vi "4Decembre2016.vi"() -> ()   [LabVIEW 2014]
panel:
  out "Partie 2 ID":i32
  out "Partie 2":string[](array[string])
  out "Partie 1":i32
  out "CharPlusLettre":string[](array[string])
  out "CharPlusNombre":i32[](array[numeric])
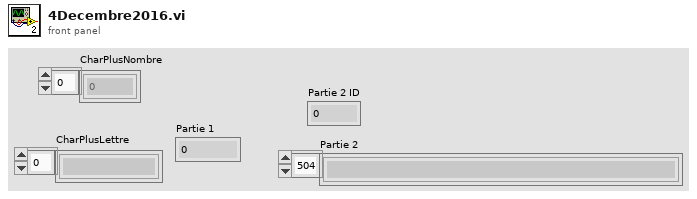
[diagram p1: front panel]
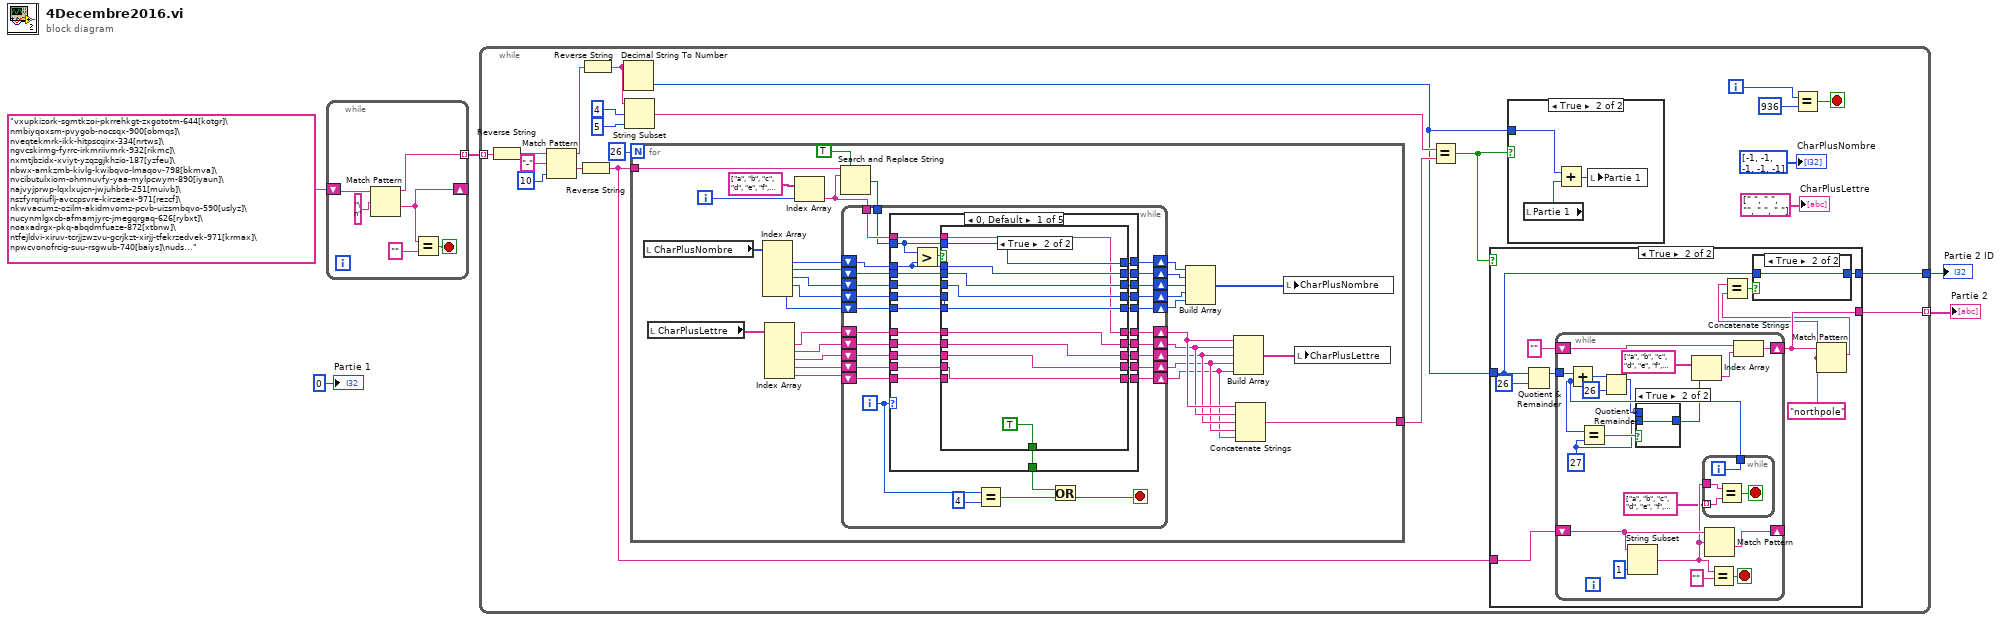
[diagram p0: block diagram]
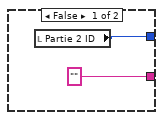
[diagram p2: hidden frame]
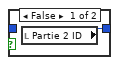
[diagram p3: hidden frame]
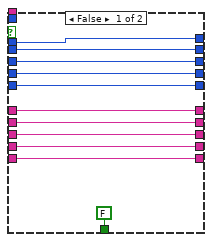
[diagram p6: hidden frame]
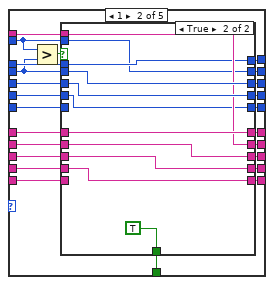
[diagram p7: hidden frame]
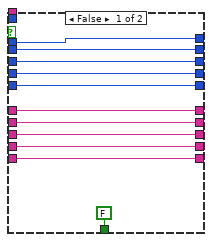
[diagram p8: hidden frame]
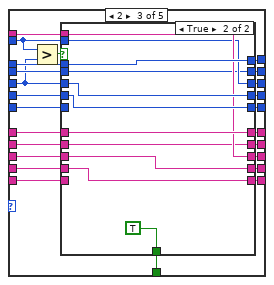
[diagram p9: hidden frame]
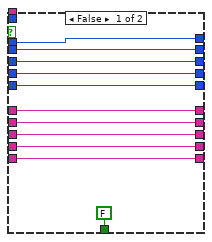
[diagram p10: hidden frame]
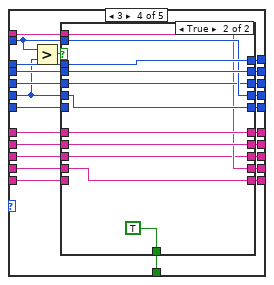
[diagram p11: hidden frame]
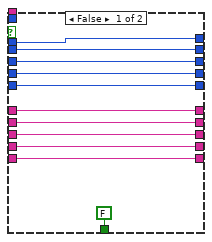
[diagram p12: hidden frame]
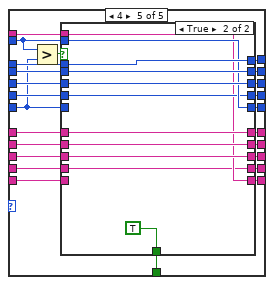
[diagram p13: hidden frame]
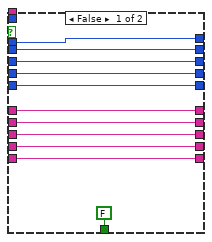
[diagram p14: hidden frame]
diagram:
  n1 = while {
    shift-right: [w8] -> _
    shift-left: "vxupkizork-sgmtkzoi-pkrrehkgt-zxgototm-644[kotgr]\nmbiyqoxsm-pvygob-nocsqx-900[obmqs]\nveqtekmrk-ikk-hitpscqirx-334[nrtws]\ngvcskirmg-fyrrc-irkmriivmrk-932[rikmc]\nxmtjbzidx-xviyt-yzqzgjkhzio-187[yzfeu]\nbwx-amkzmb-kivlg-kwibqvo-lmaqov-798[bkmva]\nvcibutulxiom-ohmnuvfy-yaa-mylpcwym-890[iyaun]\najvyjprwp-lqxlxujcn-jwjuhbrb-251[muivb]\nszfyrqriuflj-avccpsvre-kirzezex-971[rezcf]\nkwvacumz-ozilm-akidmvomz-pcvb-uizsmbqvo-590[uslyz]\nucynmlgxcb-afmamjyrc-jmegqrgaq-626[rybxt]\noaxadrgx-pkq-abqdmfuaze-872[xtbnw]\ntfejldvi-xiruv-tcrjjzwzvu-gcrjkzt-xirjj-tfekrzedvek-971[krmax]\npwcvonofrcig-suu-rsgwub-740[baiys]\nudskkaxawv-tskcwl-dgyaklauk-632[lqcfd]\nvqr-ugetgv-dcumgv-fgxgnqrogpv-258[ctwyp]\nlaffe-igtje-gtgreyoy-124[uscwl]\niehepwnu-cnwza-oywrajcan-dqjp-lqnydwoejc-368[sypjw]\nmbiyqoxsm-excdklvo-pvygob-bocokbmr-640[hslwz]\nhoungfgxjuay-pkrrehkgt-jkvruesktz-930[nsbth]\ntcfkqcevkxg-lgnnadgcp-eqpvckpogpv-388[ausbh]\nhcd-gsqfsh-wbhsfbohwcboz-pibbm-aofyshwbu-532[bhsfo]\njyfvnlupj-zjhclunly-obua-huhsfzpz-461[jopil]\npbybeshy-rtt-fgbentr-819[vxcue]\nkwtwznct-akidmvomz-pcvb-lmaqov-564[mvack]\npdjqhwlf-udeelw-uhdftxlvlwlrq-595[ldwef]\naoubshwq-gqojsbusf-vibh-gsfjwqsg-922[qfetx]\nwfintfhynaj-wfruflnsl-gzssd-ijajqturjsy-931[mkhsc]\nqspkfdujmf-kfmmzcfbo-eftjho-675[skbda]\ndmbttjgjfe-fhh-ufdiopmphz-129[nbqyz]\ntinnm-tzcksf-obozmgwg-194[mduaf]\niwcjapey-qjopwxha-ywjzu-ykwpejc-skngodkl-706[kjfog]\nkwtwznct-xzwrmkbqtm-lgm-bmkpvwtwog-356[wmtkb]\nbkwzkqsxq-wkqxodsm-mrymyvkdo-nozkbdwoxd-640[unlfi]\navb-abpfdk-185[cwyms]\nxfbqpojafe-kfmmzcfbo-vtfs-uftujoh-857[nserj]\ngsvvswmzi-jpsaiv-pefsvexsvc-516[hbidf]\ntfejldvi-xiruv-treup-kvtyefcfxp-321[mntlv]\nsxdobxkdsyxkv-mrymyvkdo-mecdywob-cobfsmo-588[emgkf]\nluxciuwncpy-vohhs-mylpcwym-292[yiojz]\nide-htrgti-hrpktcvtg-wjci-bpcpvtbtci-583[tcipb]\nsurmhfwloh-fkrfrodwh-hqjlqhhulqj-621[hflqr]\nzuv-ykixkz-yigbktmkx-natz-xkikobotm-540[zyvui]\nxmtjbzidx-wpiit-hvivbzhzio-759[kgzsj]\nmvkccspson-nio-ckvoc-666[mnklu]\nzixppfcfba-yrkkv-ildfpqfzp-991[amdtz]\nvjpwncrl-bljenwpna-qdwc-cajrwrwp-251[tgzku]\ngntmfefwitzx-xhfajsljw-mzsy-uzwhmfxnsl-671[fmswx]\najmrxjlcren-yujbcrl-pajbb-fxatbqxy-407[tszqw]\nvotubcmf-cjpibabsepvt-qmbtujd-hsbtt-nbobhfnfou-129[btfou]\netyyx-rbzudmfdq-gtms-nodqzshnmr-339[okzyu]\nbxaxipgn-vgpst-rpcsn-rdcipxcbtci-557[nmtks]\nzlilocri-oxyyfq-pxibp-939[ilopx]\nxqvwdeoh-hjj-uhvhdufk-985[uixsv]\nfrqvxphu-judgh-gbh-vhuylfhv-907[gxkts]\nrkpqxyib-oxyyfq-obpbxoze-315[jysdq]\nckgvutofkj-jek-giwaoyozout-436[tsfzu]\nzilqwikbqdm-ntwemz-lmaqov-616[mqilw]\npkl-oaynap-acc-qoan-paopejc-446[muyva]\nlxuxaodu-ajkkrc-bnaerlnb-771[yzint]\nwfruflnsl-gzssd-ijuqtdrjsy-515[zdeyi]\nmvhkvbdib-wpiit-nzmqdxzn-421[tryva]\naoubshwq-foppwh-sbuwbssfwbu-558[zhyen]\nencuukhkgf-gii-hkpcpekpi-414[kipce]\nsehheiylu-rkddo-bqrehqjeho-608[pfmot]\nirdgrxzex-avccpsvre-ivtvzmzex-529[intur]\nykhknbqh-ywjzu-klanwpekjo-784[khjnw]\ngpewwmjmih-tvsnigxmpi-fewoix-vigimzmrk-594[unmjc]\nvxupkizork-vrgyzoi-mxgyy-gtgreyoy-826[kmnot]\nqmpmxevc-kvehi-wgezirkiv-lyrx-xiglrspskc-438[gdkrm]\nixccb-fkrfrodwh-orjlvwlfv-933[nyhrz]\nlujbbrornm-ljwmh-lxjcrwp-lxwcjrwvnwc-511[wjlrc]\neqpuwogt-itcfg-ecpfa-wugt-vguvkpi-934[nchrl]\nnwlddtqtpo-mldvpe-wlmzclezcj-691[gznml]\nrdchjbtg-vgpst-rpcsn-rdpixcv-uxcpcrxcv-453[zyutx]\nwillimcpy-wuhxs-xypyfijgyhn-942[vxyeb]\nqzchnzbshud-eknvdq-rsnqzfd-521[dnqzh]\nfroruixo-mhoobehdq-rshudwlrqv-179[mbthd]\nmvydjvxodqz-nxvqzibzm-cpio-mzxzdqdib-837[yzntw]\nyknnkoera-bhksan-iwjwcaiajp-394[aknij]\nxjgjmapg-wpiit-vivgtndn-993[cyqvm]\nxgvnndadzy-xjmmjndqz-xviyt-xjvodib-gjbdnodxn-265[kgvsh]\nsbnqbhjoh-tdbwfohfs-ivou-fohjoffsjoh-467[ofcde]\ncybyjqho-whqtu-zubboruqd-tufbeocudj-842[rqply]\nbkwzkqsxq-zvkcdsm-qbkcc-nocsqx-406[xydnz]\ntinnm-foadouwbu-dzoghwq-ufogg-obozmgwg-142[rakqb]\nrdchjbtg-vgpst-rpcsn-rdpixcv-bpcpvtbtci-765[mkoez]\npinovwgz-mvwwdo-zibdizzmdib-395[smtjh]\npyknyegle-njyqrga-epyqq-bcnjmwkclr-782[yxcjz]\nvkrhzxgbv-cxeeruxtg-phkdlahi-709[tyzhs]\nudskkaxawv-vqw-vwnwdghewfl-658[wvadk]\ngsrwyqiv-kvehi-ikk-asvowlst-438[iksvw]\nlahxpnwrl-mhn-vjwjpnvnwc-173[nwhjl]\nrzvkjiduzy-ytz-xjiovdihzio-993[sumvy]\navw-zljyla-yhiipa-zhslz-825[mitza]\nudpsdjlqj-udglrdfwlyh-mhoobehdq-whfkqrorjb-673[dhjlo]\niruzfrtkzmv-wlqqp-wcfnvi-jyzggzex-841[wszry]\nrtqlgevkng-lgnnadgcp-ujkrrkpi-986[wpktr]\nktwbhtvmbox-utldxm-ftgtzxfxgm-995[uqlbn]\ndlhwvupglk-qlssfilhu-zopwwpun-149[tvkqz]\ngcfcnuls-aluxy-yaa-omyl-nymncha-292[aycln]\njrncbavmrq-enqvbnpgvir-pnaql-qrirybczrag-455[ybfie]\nfydelmwp-mfyyj-cplnbftdtetzy-613[whuxk]\nvetllbybxw-lvtoxgzxk-angm-mxvaghehzr-475[eswan]\naoubshwq-pibbm-fsoqeiwgwhwcb-662[qfaze]\niutyaskx-mxgjk-vrgyzoi-mxgyy-iayzuskx-ykxboik-722[sxnli]\nwihmogyl-aluxy-wuhxs-wiuncha-xyjulngyhn-578[pntgy]\nktiaaqnqml-kzgwomvqk-xtiabqk-oziaa-twoqabqka-226[aqkio]\nrgndvtcxr-tvv-ldgzhwde-999[tbefa]\nqyujihctyx-vcibutulxiom-wuhxs-wiuncha-xymcah-552[sdmer]\nfmsledevhsyw-fyrrc-xiglrspskc-386[yrhfz]\nqekrixmg-hci-ywiv-xiwxmrk-490[tynsr]\ngcfcnuls-aluxy-vumeyn-yhachyylcha-604[xtfeg]\niutyaskx-mxgjk-pkrrehkgt-gtgreyoy-384[gyblm]\nhmsdqmzshnmzk-rbzudmfdq-gtms-kzanqzsnqx-937[grhez]\neqttqukxg-gii-cpcnauku-362[zypxw]\nynukcajey-xekdwvwnzkqo-xqjju-odellejc-316[jglep]\nmfklstdw-uzgugdslw-lwuzfgdgyq-320[topmx]\nbuzahisl-ihzrla-zopwwpun-487[rzsag]\nvcibutulxiom-vumeyn-mylpcwym-916[tjvzx]\nmvydjvxodqz-nxvqzibzm-cpio-gjbdnodxn-733[xtcbl]\nfrqvxphu-judgh-udeelw-xvhu-whvwlqj-595[huvwd]\nfhezusjybu-tou-skijecuh-iuhlysu-608[uhsei]\nhoungfgxjuay-vrgyzoi-mxgyy-sgxqkzotm-124[mgfhr]\nodkasqzuo-uzfqdzmfuazmx-eomhqzsqd-tgzf-fqotzaxask-508[tmxza]\nfydelmwp-upwwjmply-dlwpd-873[gyzjx]\nyuxufmdk-sdmpq-dmnnuf-dqeqmdot-742[dmquf]\nxst-wigvix-fewoix-wepiw-464[mltfd]\njsehsyafy-tskcwl-dgyaklauk-190[aksyl]\nfubrjhqlf-fdqgb-uhdftxlvlwlrq-855[flqbd]\nwifilzof-xsy-mbcjjcha-422[olxnw]\nbknsykmdsfo-mrymyvkdo-nofovyzwoxd-614[oydkm]\nrtqlgevkng-hnqygt-tgceswkukvkqp-232[gkqte]\nvjpwncrl-lqxlxujcn-vjatncrwp-407[cjlnp]\nsbnqbhjoh-dpssptjwf-fhh-gjobodjoh-935[ckpbr]\nvcibutulxiom-dyffsvyuh-lyuwkocmcncih-838[flhey]\nnzydfxpc-rclop-dnlgpyrpc-sfye-opawzjxpye-899[pycde]\ndzczkrip-xiruv-treup-drerxvdvek-373[rdevi]\nryexqpqhteki-muqfedyput-isqludwuh-xkdj-qdqboiyi-244[qdiue]\nvkrhzxgbv-ktfitzbgz-vahvhetmx-vnlmhfxk-lxkobvx-735[smnif]\najvyjprwp-snuuhknjw-bqryyrwp-329[mdzxw]\nwihmogyl-aluxy-luvvcn-guhuaygyhn-188[qjwtv]\nxgvnndadzy-zbb-kpmxcvndib-395[bdnvx]\ndkqjcbctfqwu-ecpfa-eqcvkpi-ncdqtcvqta-726[paioe]\ntbxmlkfwba-avb-cfkxkzfkd-133[gmhkl]\ntfcfiwlc-gifavtkzcv-avccpsvre-cfxzjkztj-139[cusqi]\nhafgnoyr-enoovg-npdhvfvgvba-351[vgnoa]\nlzfmdshb-etyyx-cxd-rsnqzfd-547[clnoz]\nsawlkjevaz-zua-nawymqeoepekj-316[fpaeb]\npbafhzre-tenqr-pnaql-pbngvat-znexrgvat-299[iymnw]\ndmybmsuzs-nmewqf-emxqe-768[tzycl]\ndlhwvupglk-qlssfilhu-lunpullypun-695[tidnq]\nhafgnoyr-pubpbyngr-erprvivat-741[vynbz]\nodiih-mhn-jlzdrbrcrxw-459[rdhib]\ntcfkqcevkxg-tcddkv-tgugctej-986[mejtb]\nvkrhzxgbv-ietlmbv-zktll-kxtvjnblbmbhg-189[blvkt]\ngsvvswmzi-ikk-eguymwmxmsr-282[bkasy]\njqwpihizlwca-rmttgjmiv-ivitgaqa-694[eibnd]\nkzeed-jll-fsfqdxnx-697[abodg]\nxtwtelcj-rclop-prr-hzcvdsza-977[crlpt]\nnuatmlmdpage-ngzzk-dqmocgueufuaz-872[oldhw]\npybgmyargtc-pyzzgr-kylyeckclr-678[ycgrk]\nyhwooebeaz-acc-klanwpekjo-316[xmynz]\nqzlozfhmf-azrjds-vnqjrgno-781[ycnzs]\nqvbmzvibqwvit-zijjqb-bziqvqvo-252[tcfan]\nkfg-jvtivk-nvrgfezqvu-treup-cfxzjkztj-217[vfjkt]\npelbtravp-rtt-bcrengvbaf-845[evbkq]\npkl-oaynap-zua-iwngapejc-420[nkjyh]\nqekrixmg-gerhc-gsexmrk-gsrxemrqirx-490[ciuyw]\nqczcftiz-pibbm-oqeiwgwhwcb-324[kzdfm]\nfoadouwbu-qvcqczohs-gvwddwbu-454[qsnwz]\ntfiifjzmv-treup-tfekrzedvek-555[usbvt]\nnglmtuex-ietlmbv-zktll-kxtvjnblbmbhg-891[lbtme]\nixccb-fdqgb-fxvwrphu-vhuylfh-179[kesml]\nrzvkjiduzy-nxvqzibzm-cpio-mznzvmxc-941[vzopy]\nnwzekwypera-bhksan-klanwpekjo-498[kaenw]\nnjmjubsz-hsbef-tdbwfohfs-ivou-xpsltipq-571[sbfhi]\nrdchjbtg-vgpst-rdadguja-eaphixr-vgphh-tcvxcttgxcv-765[fzjti]\nxfbqpojafe-gmpxfs-vtfs-uftujoh-493[pshct]\ntcfkqcevkxg-ecpfa-tgceswkukvkqp-154[kcefg]\nhqtyeqsjylu-rkddo-huiuqhsx-530[hquds]\nqzoggwtwsr-qcffcgwjs-qvcqczohs-zcuwghwqg-246[jiwnp]\nwlqqp-sleep-ivtvzmzex-555[vsoly]\ntcfkqcevkxg-dwppa-wugt-vguvkpi-986[hcpyu]\ndpmpsgvm-xfbqpojafe-dipdpmbuf-tijqqjoh-805[wgnqv]\nksodcbwnsr-dzoghwq-ufogg-zopcfohcfm-870[dxmtj]\ntcfkqcevkxg-dcumgv-wugt-vguvkpi-856[ehozy]\nfbebmtkr-zktwx-cxeeruxtg-ftgtzxfxgm-709[tuvsx]\ndiozmivodjivg-pinovwgz-wvnfzo-rjmfncjk-863[tqdns]\nvkppo-zubboruqd-bqrehqjeho-842[qfsjm]\nmbiyqoxsm-nio-nozvyiwoxd-614[mstez]\nohmnuvfy-yaa-uhufsmcm-214[muafh]\nnzcczdtgp-ojp-afcnsldtyr-769[cdnpt]\ntinnm-xszzmpsob-fsqswjwbu-558[sbmnw]\nhwbba-uecxgpigt-jwpv-fgrnqaogpv-752[upmvg]\nmvydjvxodqz-xcjxjgvoz-jkzmvodjin-187[jvdox]\nwdjcvuvmyjpn-mvwwdo-xpnojhzm-nzmqdxz-889[mdjnv]\nbpvctixr-qjccn-sthxvc-817[ctvxb]\nrdadguja-rwdrdapit-steadnbtci-271[coqre]\nkfg-jvtivk-treup-tfrkzex-fgvirkzfej-373[sptcw]\nnbhofujd-dboez-dpbujoh-tfswjdft-493[sftdx]\nksodcbwnsr-pogysh-qighcasf-gsfjwqs-116[tvqso]\nbqvvu-ywjzu-paydjkhkcu-810[rgpzu]\ncvabijtm-lgm-zmamizkp-954[tsrpy]\nnpmhcargjc-qaytclecp-fslr-rcaflmjmew-834[lgkrj]\naflwjfslagfsd-kusnwfywj-zmfl-ksdwk-164[enmyr]\njlidywncfy-dyffsvyuh-qilembij-422[jmryi]\ndmybmsuzs-dmnnuf-dqeqmdot-586[hdgkv]\nqspkfdujmf-cbtlfu-mphjtujdt-701[zatkl]\nnvrgfezqvu-sleep-ivrthlzjzkzfe-373[udyzv]\ntbxmlkfwba-yxphbq-pqloxdb-809[tzsjm]\npelbtravp-enoovg-grpuabybtl-559[oqctv]\ndkqjcbctfqwu-ecpfa-ewuvqogt-ugtxkeg-544[cegqt]\nxgsvgmotm-xghhoz-lotgtiotm-384[gotmh]\nudskkaxawv-jsvagsulanw-kusnwfywj-zmfl-klgjsyw-346[swakj]\nkrxqjijamxdb-kjbtnc-ujkxajcxah-173[izxny]\nmyvybpev-lkcuod-nocsqx-770[yzjqg]\nupq-tfdsfu-cbtlfu-eftjho-623[ftubc]\nnpmhcargjc-qaytclecp-fslr-jmegqrgaq-444[nocrz]\niuxxuyobk-vrgyzoi-mxgyy-giwaoyozout-566[kymts]\navw-zljyla-qlssfilhu-klwhyatlua-513[tskre]\nmvhkvbdib-kmjezxodgz-agjrzm-mznzvmxc-135[suyop]\nqzlozfhmf-azrjds-dmfhmddqhmf-183[dfmhz]\nkgjgrypw-epybc-cee-qcptgacq-418[gqyos]\nguahyncw-vcibutulxiom-yaa-qilembij-968[xgtow]\nlugjuacha-wihmogyl-aluxy-wuhxs-xyjulngyhn-864[qbefr]\niehepwnu-cnwza-ykjoqian-cnwza-zua-lqnydwoejc-680[pfmiz]\nmtzslklcozfd-upwwjmply-cpdplcns-743[rngoy]\ndfcxsqhwzs-foppwh-difqvogwbu-454[fwdho]\nirdgrxzex-jtrmvexvi-ylek-nfibjyfg-139[kwabl]\njvyyvzpcl-tpspahyf-nyhkl-msvdly-ylhjxbpzpapvu-695[oyedt]\nqmpmxevc-kvehi-fewoix-qerekiqirx-282[tzsca]\nhcd-gsqfsh-suu-gozsg-870[nmehc]\nhwdtljsnh-xhfajsljw-mzsy-xytwflj-697[jhlsw]\nudpsdjlqj-iorzhu-pdunhwlqj-959[djuhl]\nenqvbnpgvir-onfxrg-svanapvat-507[nvagp]\nrzvkjiduzy-wpiit-mznzvmxc-213[ntuoi]\ngsrwyqiv-kvehi-fyrrc-xiglrspskc-776[hgnvt]\ngvaaz-cbtlfu-mbcpsbupsz-103[bacps]\nhplazytkpo-mfyyj-opawzjxpye-197[pyajo]\nraphhxuxts-gpbepvxcv-rpcsn-rdpixcv-stepgibtci-531[omniy]\ncxy-bnlanc-kdwwh-mnyuxhvnwc-251[ditcg]\nhtsxzrjw-lwfij-hmthtqfyj-yjhmstqtld-307[conpl]\nikhcxvmbex-vtgwr-lxkobvxl-345[cdftu]\nsgmtkzoi-pkrrehkgt-lotgtiotm-566[tgkoi]\ngbc-frperg-onfxrg-freivprf-455[nymsw]\nide-htrgti-hrpktcvtg-wjci-apqdgpidgn-531[gitdp]\ndpmpsgvm-gmpxfs-tupsbhf-259[hgopn]\nxmrrq-kusnwfywj-zmfl-wfyafwwjafy-892[fwyaj]\nqfmcusbwq-tinnm-pogysh-rsdzcmasbh-428[bgfat]\nzhdsrqlchg-lqwhuqdwlrqdo-vfdyhqjhu-kxqw-ghyhorsphqw-803[smjtn]\ncrwwv-pzxsbkdbo-erkq-pxibp-601[tnzmy]\nxgjougizobk-jek-jkvruesktz-592[wsdmo]\nbnqqnrhud-okzrshb-fqzrr-cdozqsldms-963[jtram]\nqjopwxha-fahhuxawj-qoan-paopejc-472[ahjop]\namppmqgtc-amjmpdsj-afmamjyrc-kylyeckclr-184[yxzuq]\nthnulapj-ihzrla-mpuhujpun-643[uhpaj]\nlzfmdshb-oqnidbshkd-rbzudmfdq-gtms-btrsnldq-rdquhbd-833[dbqsh]\nnzwzcqfw-mldvpe-cpdplcns-119[sejuv]\niqmbazulqp-omzpk-oamfuzs-dqeqmdot-950[qylkj]\nlxaaxbren-lqxlxujcn-mnyuxhvnwc-849[frqsy]\nnzwzcqfw-xtwtelcj-rclop-nlyoj-nzletyr-xlylrpxpye-743[lycen]\nfubrjhqlf-sodvwlf-judvv-rshudwlrqv-621[ghonw]\niuxxuyobk-yigbktmkx-natz-ygrky-514[meayn]\nwkqxodsm-nio-myxdksxwoxd-692[rqmey]\njvuzbtly-nyhkl-jvsvymbs-msvdly-klwsvftlua-305[yxmzb]\nwlqqp-wcfnvi-uvmvcfgdvek-581[xriqe]\nqcffcgwjs-tzcksf-fsqswjwbu-116[ztnym]\nlahxpnwrl-kdwwh-mnenuxyvnwc-719[nwhlx]\nmuqfedyput-cqwdujys-fbqijys-whqii-mehaixef-634[iqefu]\neqpuwogt-itcfg-ejqeqncvg-gpikpggtkpi-232[kzfyv]\niwcjapey-xwogap-lqnydwoejc-420[styzx]\ntagzsrsjvgmk-jsttal-mkwj-lwklafy-502[nrteu]\nfrqvxphu-judgh-udeelw-sxufkdvlqj-725[hzbtv]\nkzgwomvqk-kivlg-kwibqvo-uizsmbqvo-746[epcdb]\nckgvutofkj-pkrrehkgt-ygrky-696[yblnm]\nydjuhdqjyedqb-vbemuh-tuiywd-894[oybua]\ndwbcjkun-mhn-bjunb-121[srjlk]\nejpanjwpekjwh-qjopwxha-acc-qoan-paopejc-290[bsjiz]\nirgyyolokj-inuiurgzk-xkgiwaoyozout-774[oigku]\nmfklstdw-xdgowj-vwhsjlewfl-320[xyfdh]\nsawlkjevaz-xwogap-klanwpekjo-420[mpkso]\nfbebmtkr-zktwx-vhehkyne-lvtoxgzxk-angm-vnlmhfxk-lxkobvx-241[kxvbe]\nirdgrxzex-vxx-glityrjzex-893[sxqom]\nhqtyeqsjylu-rkddo-cqhaujydw-946[gastx]\nlujbbrornm-kjbtnc-bjunb-251[xazbt]\niehepwnu-cnwza-bhksan-zarahkliajp-680[hlqnu]\nxcjxjgvoz-vivgtndn-629[yubnv]\nixeumktoi-lruckx-sgtgmksktz-332[mrldq]\nqxdwpopgsdjh-rpcsn-rdpixcv-ldgzhwde-765[rxoey]\nglrcplyrgmlyj-njyqrga-epyqq-pcacgtgle-158[stgxu]\nojk-nzxmzo-kgvnodx-bmvnn-nzmqdxzn-525[nzmox]\nfroruixo-mhoobehdq-fxvwrphu-vhuylfh-933[ycnsx]\nhdgdovmt-bmvyz-wvnfzo-omvdidib-395[hdygz]\naczupnetwp-ncjzrpytn-nlyoj-nzletyr-ecltytyr-535[ntyce]\nfnjyxwrinm-ajkkrc-cajrwrwp-537[nczta]\nrgllk-gzefmnxq-omzpk-oamfuzs-fqotzaxask-300[ztbqp]\nmuqfedyput-sqdto-fkhsxqiydw-218[npsrc]\nbuzahisl-jovjvshal-jvuahputlua-747[lsatz]\niuruxlar-lruckx-sgtgmksktz-826[krugl]\nthnulapj-jovjvshal-ylzlhyjo-513[mtegl]\njshzzpmplk-lnn-shivyhavyf-201[hlnps]\nqekrixmg-jpsaiv-pefsvexsvc-646[ryhkz]\nmhi-lxvkxm-unggr-kxlxtkva-163[fkcax]\nlugjuacha-wbiwifuny-wihnuchgyhn-396[huinw]\nsbejpbdujwf-tdbwfohfs-ivou-tfswjdft-545[pnmzi]\nnwilwcejc-zua-bejwjyejc-524[jcewa]\nxlrypetn-awldetn-rcldd-xlcvpetyr-249[jgkyr]\namlqskcp-epybc-bwc-pcacgtgle-990[iyqge]\nktfitzbgz-lvtoxgzxk-angm-ybgtgvbgz-761[gtzbk]\navw-zljyla-ihzrla-huhsfzpz-253[banhu]\npualyuhapvuhs-ihzrla-ylhjxbpzpapvu-903[xsuvo]\nqfkkj-nlyoj-xlcvpetyr-587[jklyc]\niruzfrtkzmv-irsszk-rthlzjzkzfe-451[zrkfi]\niqmbazulqp-vqxxknqmz-pqbxakyqzf-534[qxzab]\nudskkaxawv-kusnwfywj-zmfl-ljsafafy-892[afksw]\ngzefmnxq-ngzzk-etubbuzs-118[yjzkl]\nmolgbzqfib-ciltbo-zlkqxfkjbkq-809[isjze]\nrnqnyfwd-lwfij-ojqqdgjfs-wjhjnansl-671[jnfqw]\nfruurvlyh-ixccb-exqqb-uhfhlylqj-751[hlqub]\npinovwgz-zbb-nvgzn-343[sdhnt]\njoufsobujpobm-dipdpmbuf-eftjho-181[ltrqy]\nqzchnzbshud-rbzudmfdq-gtms-bnmszhmldms-209[seypq]\nxfbqpojafe-dboez-sftfbsdi-649[fbdeo]\nqjopwxha-ywjzu-zalhkuiajp-238[diyme]\nocipgvke-ecpfa-gpikpggtkpi-310[moyvi]\nlxwbdvna-pajmn-vjpwncrl-bljenwpna-qdwc-vjwjpnvnwc-589[pvqom]\nglrcplyrgmlyj-zyqicr-pcacgtgle-964[djtcm]\nckgvutofkj-kmm-jkbkruvsktz-254[twvxe]\npyknyegle-bwc-bcnyprkclr-522[oktmn]\namjmpdsj-zyqicr-asqrmkcp-qcptgac-314[campq]\nqvbmzvibqwvit-akidmvomz-pcvb-zmamizkp-902[zvsto]\nvxupkizork-igtje-iugzotm-jkvruesktz-748[bvyza]\nkpvgtpcvkqpcn-dcumgv-wugt-vguvkpi-596[znbmg]\nzovldbkfz-ciltbo-abmxoqjbkq-705[tknsq]\ntagzsrsjvgmk-xdgowj-jwuwanafy-476[agjws]\nmrxivrexmsrep-glsgspexi-hitevxqirx-256[atzwx]\npelbtravp-enoovg-znantrzrag-195[wdneq]\nocipgvke-eqttqukxg-dcumgv-ugtxkegu-102[soynm]\neqnqthwn-ejqeqncvg-tgugctej-908[zkyam]\nhwbba-tcddkv-ocpcigogpv-206[vadln]\naflwjfslagfsd-tmffq-ogjckzgh-528[fgajl]\nnij-mywlyn-zotts-luvvcn-jolwbumcha-838[lncjm]\njvsvymbs-zjhclunly-obua-zhslz-409[bpesx]\nwfintfhynaj-hfsid-htfynsl-htsyfnsrjsy-359[ozaby]\nnzcczdtgp-upwwjmply-dpcgtnpd-795[pcdgn]\nexcdklvo-lkcuod-bomosfsxq-978[kczes]\nmrxivrexmsrep-fmsledevhsyw-ikk-vieguymwmxmsr-516[mersi]\nwillimcpy-yaa-mylpcwym-864[iucxs]\nnsyjwsfyntsfq-hfsid-btwpxmtu-957[miqnp]\njvsvymbs-kfl-klzpnu-149[tyzxi]\namlqskcp-epybc-aylbw-amyrgle-bcnjmwkclr-730[ytmsd]\nbkwzkqsxq-nio-cdybkqo-562[anfrp]\nide-htrgti-rpcsn-rdpixcv-rdcipxcbtci-635[zcbyd]\naflwjfslagfsd-tmffq-jwkwsjuz-606[fjswa]\nfoadouwbu-foppwh-oqeiwgwhwcb-714[toynm]\nnzydfxpc-rclop-prr-dezclrp-795[tszpi]\nmfklstdw-jsttal-ksdwk-944[autpj]\njvsvymbs-jhukf-zlycpjlz-409[borjv]\nlnkfaypeha-ydkykhwpa-zalwnpiajp-342[twaxy]\npbybeshy-cynfgvp-tenff-npdhvfvgvba-741[fvbnp]\nshoewudys-uww-tufbeocudj-764[iacnf]\niutyaskx-mxgjk-jek-giwaoyozout-566[koagi]\nxcitgcpixdcpa-eaphixr-vgphh-hpath-401[xwtyn]\ndlhwvupglk-wshzapj-nyhzz-lunpullypun-643[atizk]\njlidywncfy-mwupyhayl-bohn-mbcjjcha-214[wgcya]\neqpuwogt-itcfg-fag-qrgtcvkqpu-960[gqtcf]\nfab-eqodqf-eomhqzsqd-tgzf-eqdhuoqe-950[zoeyv]\noazegyqd-sdmpq-nmewqf-pqhqxabyqzf-872[pkotu]\nhqtyeqsjylu-uww-qsgkyiyjyed-946[yqejs]\npejji-mrymyvkdo-bomosfsxq-614[mojsy]\ngzefmnxq-omzpk-xasuefuoe-378[iutjy]\nhjgbwuladw-uzgugdslw-ksdwk-840[wdguk]\nkpvgtpcvkqpcn-gii-ujkrrkpi-674[juebo]\nencuukhkgf-gii-ugtxkegu-258[gukei]\nxcitgcpixdcpa-eaphixr-vgphh-rdcipxcbtci-167[pkozr]\ngcfcnuls-aluxy-wuhxs-wiuncha-lyuwkocmcncih-526[cuhln]\ndmbttjgjfe-gmpxfs-mphjtujdt-441[jtmdf]\ntcfkqcevkxg-hnqygt-tgceswkukvkqp-154[jgnim]\nxqvwdeoh-udeelw-uhdftxlvlwlrq-309[swfid]\nnzwzcqfw-ojp-wzrtdetnd-665[wzdnt]\nshoewudys-sqdto-seqjydw-iqbui-816[zyxmn]\ngzefmnxq-rxaiqd-mzmxkeue-300[cxpzy]\nsawlkjevaz-zua-zarahkliajp-472[azjkl]\nktfitzbgz-ietlmbv-zktll-lxkobvxl-345[zgpbs]\ncjpibabsepvt-gvaaz-cvooz-sftfbsdi-857[absvc]\neqpuwogt-itcfg-gii-ceswkukvkqp-128[rykin]\ntbxmlkfwba-ciltbo-pqloxdb-653[yaqrn]\nqzchnzbshud-okzrshb-fqzrr-dmfhmddqhmf-495[shpge]\ndszphfojd-upq-tfdsfu-gmpxfs-pqfsbujpot-129[tefni]\naietsrmdih-ikk-hitpscqirx-100[ihkrs]\nykhknbqh-ywjzu-ykwpejc-qoan-paopejc-992[mgfrs]\noxmeeuruqp-eomhqzsqd-tgzf-ogefayqd-eqdhuoq-768[dsutf]\nnwzekwypera-ywjzu-ykwpejc-yqopkian-oanreya-134[yaewk]\netyyx-idkkxadzm-zmzkxrhr-807[kxzdm]\nkgjgrypw-epybc-aylbw-amyrgle-bcnyprkclr-418[yrbcg]\nslqryzjc-njyqrga-epyqq-ylyjwqgq-418[saunh]\nnuatmlmdpage-qss-xasuefuoe-794[rtesp]\njvuzbtly-nyhkl-msvdly-wbyjohzpun-617[gjidl]\nbkzrrhehdc-azrjds-trdq-sdrshmf-417[dregf]\njqwpihizlwca-akidmvomz-pcvb-bmkpvwtwog-122[dywqz]\ngntmfefwitzx-idj-jslnsjjwnsl-463[xcwpd]\nmyvybpev-bkllsd-domrxyvyqi-978[otdny]\nqlm-pbzobq-pzxsbkdbo-erkq-xkxivpfp-263[jfzsm]\nlujbbrornm-kdwwh-jwjuhbrb-953[svzbm]\ndwbcjkun-yaxsnlcrun-ajkkrc-mnyuxhvnwc-303[lntzx]\nfroruixo-sodvwlf-judvv-ghvljq-595[ghbyq]\nhjgbwuladw-ugjjgkanw-xdgowj-vwhsjlewfl-944[jiyqa]\negdytrixat-gpbepvxcv-qjccn-itrwcdadvn-687[xdpsn]\nszfyrqriuflj-jtrmvexvi-ylek-uvgrikdvek-477[vbldh]\nuzfqdzmfuazmx-pkq-dqmocgueufuaz-352[owbht]\nrnqnyfwd-lwfij-gntmfefwitzx-gzssd-qfgtwfytwd-905[fwtdg]\nykhknbqh-xqjju-odellejc-498[yuzlk]\ndwbcjkun-ouxfna-bqryyrwp-485[bnruw]\neqttqukxg-etaqigpke-tcddkv-ceswkukvkqp-492[muprn]\njvyyvzpcl-ibuuf-zlycpjlz-487[imbad]\nudglrdfwlyh-gbh-whfkqrorjb-127[fvnah]\nytu-xjhwjy-jll-yjhmstqtld-385[zmyui]\nyhwooebeaz-bhksan-wymqeoepekj-316[eoabh]\nbnmrtldq-fqzcd-qzaahs-sqzhmhmf-755[jmrin]\nshoewudys-rkddo-skijecuh-iuhlysu-530[homtc]\npbeebfvir-enoovg-fuvccvat-663[fpume]\ndwbcjkun-mhn-mnbrpw-173[wscyp]\ndpmpsgvm-sbccju-nbobhfnfou-987[nmzgw]\neqnqthwn-ecpfa-eqcvkpi-gpikpggtkpi-986[pegik]\nnpmhcargjc-aylbw-bcnjmwkclr-288[xfyca]\nqfkkj-mfyyj-dezclrp-301[pdsrv]\nhmsdqmzshnmzk-dff-nodqzshnmr-859[mdhns]\ncjpibabsepvt-sbccju-bobmztjt-831[sxhat]\noaddaeuhq-omzpk-oamfuzs-dqeqmdot-586[doamq]\nqyujihctyx-luvvcn-mbcjjcha-864[pihao]\nwihmogyl-aluxy-wuhxs-zchuhwcha-578[meoti]\nszfyrqriuflj-upv-jyzggzex-867[hstwn]\nsorozgxe-mxgjk-xghhoz-ygrky-930[avuox]\njvsvymbs-yhtwhnpun-lnn-ylzlhyjo-903[yzoki]\nhcd-gsqfsh-qcbgiasf-ufors-qobrm-difqvogwbu-350[ukbjs]\nsawlkjevaz-xwogap-bejwjyejc-654[blmwy]\nqyujihctyx-jfumncw-alumm-mbcjjcha-838[cthpi]\ngvaaz-cbtlfu-efqbsunfou-649[fuabc]\nnjmjubsz-hsbef-dipdpmbuf-dvtupnfs-tfswjdf-805[dvpoe]\ndlhwvupglk-wshzapj-nyhzz-vwlyhapvuz-461[jimak]\namppmqgtc-aylbw-amyrgle-pcyaosgqgrgml-314[gamlp]\npyknyegle-afmamjyrc-nspafyqgle-860[yaefg]\njoufsobujpobm-dipdpmbuf-sfdfjwjoh-779[dnsfo]\nsorozgxe-mxgjk-ixeumktoi-inuiurgzk-zkinturume-488[nupts]\njqwpihizlwca-rmttgjmiv-camz-bmabqvo-122[ybtzv]\nhmsdqmzshnmzk-eknvdq-dmfhmddqhmf-469[tdmly]\nxgvnndadzy-agjrzm-nzmqdxzn-655[bjpti]\nkdijqrbu-fbqijys-whqii-tufbeocudj-790[mvwqd]\nzvyvgnel-tenqr-pnaql-npdhvfvgvba-481[bscyz]\nkyelcrga-zsllw-qrmpyec-106[sjnmi]\ngpewwmjmih-glsgspexi-pskmwxmgw-464[esxzf]\nrdadguja-gpqqxi-jhtg-ithixcv-973[snzut]\nvkrhzxgbv-xzz-vnlmhfxk-lxkobvx-371[qrtko]\nykjoqian-cnwza-zua-iwjwcaiajp-550[aijwc]\ngsvvswmzi-gerhc-gsexmrk-jmrergmrk-516[mdrpu]\niuruxlar-hgyqkz-xkikobotm-930[kioru]\nnij-mywlyn-yaa-nluchcha-214[wdicr]\nsbejpbdujwf-dboez-dpbujoh-efwfmpqnfou-597[yxwam]\nwlsiayhcw-mwupyhayl-bohn-xyjulngyhn-396[nmstq]\nvqr-ugetgv-ejqeqncvg-nqikuvkeu-466[eqvgu]\nyhwooebeaz-acc-iwjwcaiajp-446[acwei]\nwbhsfbohwcboz-dzoghwq-ufogg-fsoqeiwgwhwcb-610[wobgh]\nvxupkizork-igtje-uvkxgzouty-384[stomh]\nbxaxipgn-vgpst-rpcsn-sthxvc-219[pkyzm]\noxmeeuruqp-omzpk-oamfuzs-etubbuzs-534[fmryb]\nenzcntvat-rtt-ernpdhvfvgvba-819[tvnae]\nlxwbdvna-pajmn-yujbcrl-pajbb-mnyuxhvnwc-121[qonxs]\nkzeed-hmthtqfyj-wjxjfwhm-463[gisbv]\namjmpdsj-njyqrga-epyqq-rpyglgle-444[wyviq]\nftzgxmbv-utldxm-ltexl-241[ltxmb]\nlxuxaodu-lxaaxbren-bljenwpna-qdwc-mnenuxyvnwc-745[yustq]\nrwcnawjcrxwju-snuuhknjw-cnlqwxuxph-433[bzwvn]\niutyaskx-mxgjk-hgyqkz-xkikobotm-956[tvyep]\ngsrwyqiv-kvehi-nippcfier-xiglrspskc-542[iprsc]\ndiozmivodjivg-xcjxjgvoz-hvivbzhzio-265[pdjnm]\ndszphfojd-fhh-mbcpsbupsz-493[hpsbd]\nqxdwpopgsdjh-eaphixr-vgphh-stktadebtci-323[mayxe]\npelbtravp-rtt-erprvivat-897[rtpva]\nmvydjvxodqz-agjrzm-yzkvmohzio-369[nmwjo]\nuqtqbizg-ozilm-zijjqb-lmxizbumvb-200[bizmq]\ngvaaz-fhh-usbjojoh-675[ziyxw]\nygcrqpkbgf-fag-ewuvqogt-ugtxkeg-336[gefkq]\neadalsjq-yjsvw-vqw-vwhsjlewfl-294[yjmzc]\nvagreangvbany-fpniratre-uhag-npdhvfvgvba-299[ybzws]\natyzghrk-xghhoz-iutzgotsktz-436[pxlky]\nuwtojhynqj-hfsid-htfynsl-wjfhvznxnynts-229[nhfjs]\nudskkaxawv-tmffq-kzahhafy-658[afkhd]\njvuzbtly-nyhkl-wshzapj-nyhzz-shivyhavyf-591[taisq]\nnwzekwypera-xwogap-nawymqeoepekj-862[aiknj]\ngsrwyqiv-kvehi-gerhc-tyvglewmrk-490[emcda]\nbdavqofuxq-dmnnuf-mzmxkeue-924[stnrq]\ncxy-bnlanc-ljwmh-lxjcrwp-jwjuhbrb-199[jbclw]\nryexqpqhteki-uww-iqbui-972[whlao]\nguahyncw-zfiqyl-mylpcwym-292[hakyd]\nmybbycsfo-tovvilokx-wkbuodsxq-640[pwdms]\nsehheiylu-sxesebqju-cqdqwucudj-166[dqtmn]\nemixwvqhml-ntwemz-bziqvqvo-512[mqvei]\nwillimcpy-wuhxs-yhachyylcha-136[wmdkg]\naietsrmdih-jpsaiv-wlmttmrk-802[pndyu]\nxst-wigvix-veffmx-irkmriivmrk-854[vzbjm]\ndpmpsgvm-dboez-dpbujoh-dvtupnfs-tfswjdf-831[nzcoy]\nwlqqp-irsszk-rercpjzj-815[bjyfk]\nkyelcrga-aylbw-amyrgle-sqcp-rcqrgle-730[engxw]\nghkmaihex-hucxvm-lmhktzx-501[hmxka]\nbgmxkgtmbhgte-cxeeruxtg-ftkdxmbgz-449[gtxbe]\nudglrdfwlyh-iorzhu-vklsslqj-751[ldhrs]\nfmsledevhsyw-fewoix-asvowlst-282[sewfl]\nqfkkj-ojp-cpdplcns-197[yovpm]\nejpanjwpekjwh-iwcjapey-xwogap-zalwnpiajp-108[reijs]\nfoadouwbu-tzcksf-rsdzcmasbh-428[sabcd]\njyddc-gerhc-gsexmrk-erepcwmw-308[cghmn]\nynukcajey-zua-yqopkian-oanreya-732[aynek]\nzotts-vumeyn-guleyncha-968[entuy]\nenzcntvat-jrncbavmrq-rtt-fgbentr-871[htygn]\nqfkkj-dnlgpyrpc-sfye-dezclrp-353[pcdef]\nkzeed-htsxzrjw-lwfij-gzssd-tujwfyntsx-879[pefzg]\ngvcskirmg-nippcfier-vieguymwmxmsr-646[zsigf]\nncjzrpytn-nlyoj-hzcvdsza-587[tnijv]\nfkqbokxqflkxi-ciltbo-ixyloxqlov-991[tdoma]\ntagzsrsjvgmk-uzgugdslw-jwsuimakalagf-814[fzilb]\nydjuhdqjyedqb-vbemuh-tufbeocudj-764[vyuwb]\nglrcplyrgmlyj-cee-kypicrgle-574[znbys]\nfhezusjybu-sqdto-ixyffydw-244[istpq]\nwillimcpy-luvvcn-omyl-nymncha-110[lcmny]\nujoon-ytaanqtpc-jhtg-ithixcv-661[nhrwm]\naoubshwq-qobrm-ghcfous-116[ixtcr]\ngcfcnuls-aluxy-vohhs-xyjfisgyhn-526[emins]\nuiovmbqk-zijjqb-abwziom-382[ymdir]\nubhatstkwhnl-unggr-lmhktzx-371[zskyt]\ntagzsrsjvgmk-vqw-klgjsyw-476[nzitq]\nlejkrscv-wcfnvi-wzeretzex-451[tefwa]\nmyxcewob-qbkno-mkxni-oxqsxoobsxq-302[ayius]\ntagzsrsjvgmk-usfvq-ljsafafy-242[safgj]\nfab-eqodqf-dmnnuf-geqd-fqefuzs-898[igqxs]\nmtzslklcozfd-dnlgpyrpc-sfye-dezclrp-639[edrfn]\naoubshwq-gqojsbusf-vibh-fsqswjwbu-376[qpxwo]\noaxadrgx-eomhqzsqd-tgzf-pqbxakyqzf-508[qaxzd]\nluxciuwncpy-dyffsvyuh-mufym-682[kpftu]\nhcd-gsqfsh-rms-qcbhowbasbh-168[utywx]\neqpuwogt-itcfg-hnqygt-ceswkukvkqp-882[scpud]\nkfg-jvtivk-treup-drerxvdvek-841[sjpfi]\njrncbavmrq-vagreangvbany-onfxrg-ynobengbel-585[nabgr]\ntcrjjzwzvu-treup-tfrkzex-wzeretzex-113[jacik]\nnzydfxpc-rclop-clxalrtyr-mldvpe-wlmzclezcj-535[jwvqg]\ncybyjqho-whqtu-tou-kiuh-juijydw-816[zvfwe]\nhmsdqmzshnmzk-atmmx-cdoknxldms-365[mdshk]\nrgndvtcxr-eaphixr-vgphh-itrwcdadvn-947[nbcsm]\nmbggf-wshzapj-nyhzz-mpuhujpun-175[lekij]\niuruxlar-yigbktmkx-natz-sgxqkzotm-306[pkfsv]\nnsyjwsfyntsfq-kqtbjw-fsfqdxnx-203[fsnqj]\noknkvcta-itcfg-fag-rwtejcukpi-986[gszvj]\nnuatmlmdpage-dmnnuf-qzsuzqqduzs-170[udmnq]\nwlqqp-irsszk-ljvi-kvjkzex-659[kijlq]\npualyuhapvuhs-jovjvshal-jvuahputlua-513[dtigq]\nyaxsnlcrun-ajmrxjlcren-mhn-ydalqjbrwp-381[axybh]\nykhknbqh-oywrajcan-dqjp-odellejc-732[zmhol]\nzekvierkzferc-sleep-jyzggzex-867[xdzch]\nfab-eqodqf-nmewqf-oazfmuzyqzf-196[ivrwp]\ndpmpsgvm-cvooz-efqmpznfou-311[cdzpy]\nawzwhofm-ufors-xszzmpsob-difqvogwbu-272[vxzrc]\nlxwbdvna-pajmn-ljwmh-lxjcrwp-bcxajpn-173[rmdts]\nyhwooebeaz-ejpanjwpekjwh-zua-owhao-810[sreak]\nmuqfedyput-tou-fkhsxqiydw-582[udfqt]\nglrcplyrgmlyj-njyqrga-epyqq-qcptgacq-756[rlowk]\ncjpibabsepvt-joufsobujpobm-cvooz-efqmpznfou-493[wfzrg]\nvrurcjah-pajmn-snuuhknjw-nwprwnnarwp-927[nrwaj]\nsgmtkzoi-vrgyzoi-mxgyy-yzuxgmk-384[wdglh]\neadalsjq-yjsvw-tskcwl-vwhsjlewfl-294[umvwa]\npdjqhwlf-froruixo-iorzhu-vhuylfhv-985[wqsva]\nqczcftiz-dzoghwq-ufogg-obozmgwg-948[ayqfz]\ndlhwvupglk-ibuuf-shivyhavyf-227[huvfi]\nsurmhfwloh-iorzhu-ghyhorsphqw-959[horsu]\nuzfqdzmfuazmx-omzpk-etubbuzs-222[jbtnq]\nyhkpvhjapcl-jovjvshal-zlycpjlz-903[nhtyz]\nwfintfhynaj-hfsid-htfynsl-xjwanhjx-723[fhnja]\nenqvbnpgvir-pnaql-pbngvat-erfrnepu-533[nperv]\nfrqvxphu-judgh-edvnhw-frqwdlqphqw-205[hvwrq]\nirdgrxzex-irsszk-ljvi-kvjkzex-139[ikrxz]\nsorozgxe-mxgjk-vxupkizork-hatte-jkvgxzsktz-306[zieyv]\nqyujihctyx-wbiwifuny-guhuaygyhn-604[yoszc]\nlxuxaodu-npp-mnenuxyvnwc-953[wtfho]\nmyxcewob-qbkno-nio-crszzsxq-250[obcnq]\ndpotvnfs-hsbef-kfmmzcfbo-tbmft-831[nzqmy]\noxaflxzqfsb-oxyyfq-cfkxkzfkd-783[fxkoq]\nipvohghykvbz-kfl-jvuahputlua-851[huvak]\nbuzahisl-jhukf-jvhapun-hjxbpzpapvu-227[ylznv]\nnsyjwsfyntsfq-hfsid-htfynsl-yjhmstqtld-879[pdujv]\nxfbqpojafe-dipdpmbuf-vtfs-uftujoh-181[ujbvm]\nujqgywfau-ugjjgkanw-usfvq-vwhdgqewfl-450[aczqr]\nhafgnoyr-rtt-znantrzrag-481[qyxab]\novbunmneqbhf-rtt-qrirybczrag-897[rbnqt]\nvcibutulxiom-jfumncw-alumm-nywbhifias-318[angjx]\nluxciuwncpy-yaa-uhufsmcm-344[eupia]\ncrwwv-oxaflxzqfsb-yxphbq-abmxoqjbkq-679[bqxaf]\nrdchjbtg-vgpst-hrpktcvtg-wjci-ejgrwphxcv-557[gmont]\navw-zljyla-jhukf-ylzlhyjo-617[xmgat]\nfydelmwp-awldetn-rcldd-xlylrpxpye-691[umlsi]\namppmqgtc-njyqrga-epyqq-pcqcypaf-522[jmnui]\nkmjezxodgz-nxvqzibzm-cpio-omvdidib-135[jifak]\nkzgwomvqk-jiasmb-bziqvqvo-616[nxhic]\nlxuxaodu-ljwmh-mnyuxhvnwc-303[ekywx]\nbwx-amkzmb-kpwkwtibm-uiviomumvb-200[fopng]\nyknnkoera-xqjju-nayaerejc-238[imwko]\nwlsiayhcw-wifilzof-xsy-lymyulwb-604[lwyif]\ntvsnigxmpi-gerhc-gsexmrk-pskmwxmgw-230[dlhtu]\npinovwgz-xcjxjgvoz-adivixdib-343[pmnjr]\nlnkfaypeha-xwogap-skngodkl-888[hwxrv]\ntvsnigxmpi-hci-asvowlst-568[lrakt]\ntipfxvezt-treup-rercpjzj-191[bxghm]\nnzydfxpc-rclop-nlyoj-wzrtdetnd-483[xvftz]\nbnmrtldq-fqzcd-azrjds-kzanqzsnqx-391[ketyf]\nzekvierkzferc-sleep-kirzezex-477[otfzl]\nxfbqpojafe-nbhofujd-sbccju-bobmztjt-649[bjfoc]\nlgh-kwujwl-hdsklau-yjskk-ljsafafy-320[nzyav]\neqpuwogt-itcfg-ejqeqncvg-yqtmujqr-440[dmpcx]\namlqskcp-epybc-bwc-dglylagle-834[oqwzc]\nhvbizodx-kgvnodx-bmvnn-gvwjmvojmt-603[gheqr]\nbuzahisl-msvdly-zlycpjlz-227[urzfe]\ngvaaz-kfmmzcfbo-bdrvjtjujpo-207[jabfm]\nnzcczdtgp-qwzhpc-dezclrp-197[czpde]\ngsvvswmzi-veffmx-viwievgl-386[znley]\ndyz-combod-mkxni-crszzsxq-354[xymnl]\nzuv-ykixkz-pkrrehkgt-iutzgotsktz-748[ktzgi]\nrgndvtcxr-eaphixr-vgphh-tcvxcttgxcv-531[pntam]\nqfmcusbwq-foppwh-rsjszcdasbh-662[sbcfh]\nvdzonmhydc-dff-zmzkxrhr-391[pkeyc]\nclxalrtyr-mldvpe-nzyeltyxpye-353[dmtcw]\nxgjougizobk-inuiurgzk-zkinturume-254[hqutr]\nlsyrkjkbnyec-lkcuod-nocsqx-172[axnjt]\noxjmxdfkd-pzxsbkdbo-erkq-jxohbqfkd-965[dmnfi]\nrkpqxyib-yxphbq-zrpqljbo-pbosfzb-471[bpqor]\nglrcplyrgmlyj-bwc-pcqcypaf-262[clpyg]\nmybbycsfo-nio-psxkxmsxq-432[znbfc]\nfubrjhqlf-vfdyhqjhu-kxqw-ghvljq-257[xygze]\najvyjprwp-ajkkrc-vjwjpnvnwc-667[jpvwa]\nqfmcusbwq-rms-obozmgwg-740[tjyop]\nxlrypetn-mldvpe-nzyeltyxpye-171[jyfxu]\nzlkprjbo-doxab-mixpqfz-doxpp-xznrfpfqflk-809[icbft]\nvjpwncrl-lqxlxujcn-mnyuxhvnwc-407[sygbx]\nwlqqp-treup-tfrkzex-uvjzxe-815[rnolz]\nahngzyzqcntr-idkkxadzm-lzqjdshmf-183[zdahk]\nmrxivrexmsrep-jpsaiv-asvowlst-594[ldpzc]\njsvagsulanw-wyy-wfyafwwjafy-918[plqyr]\nixeumktoi-yigbktmkx-natz-aykx-zkyzotm-436[ergam]\npybgmyargtc-njyqrga-epyqq-nspafyqgle-782[ushvj]\nkfg-jvtivk-wcfnvi-jrcvj-919[vjcfi]\nfubrjhqlf-ixccb-iorzhu-uhvhdufk-309[qkwnm]\nmuqfedyput-fbqijys-whqii-mehaixef-400[shvuf]\ntcrjjzwzvu-avccpsvre-jyzggzex-685[fyzub]\nzgmfyxypbmsq-zyqicr-bcnjmwkclr-938[utmil]\nhoungfgxjuay-pkrrehkgt-yzuxgmk-488[xszwt]\npbeebfvir-pnaql-erprvivat-247[vhuxi]\nqvbmzvibqwvit-kpwkwtibm-abwziom-694[rnmtq]\nmvhkvbdib-zbb-pnzm-oznodib-395[ldmui]\nqxdwpopgsdjh-rwdrdapit-stktadebtci-245[dtpai]\nxgsvgmotm-lruckx-sgtgmksktz-514[nestp]\nmuqfedyput-zubboruqd-huiuqhsx-738[uqbdh]\nlaffe-hatte-lotgtiotm-566[taefl]\nrdchjbtg-vgpst-rpcsn-hidgpvt-921[gptcd]\nnwilwcejc-nwxxep-zarahkliajp-160[awcei]\njvyyvzpcl-jyfvnlupj-zjhclunly-obua-ayhpupun-929[zcymu]\ngbc-frperg-cynfgvp-tenff-nanylfvf-429[pszmb]\nnzwzcqfw-qwzhpc-xlcvpetyr-587[qmjln]\nucynmlgxcb-zyqicr-jmegqrgaq-730[cgqmr]\ngbc-frperg-sybjre-grpuabybtl-351[giufw]\nhqcfqwydw-hqrryj-mehaixef-608[hqefr]\nyflexwxoalrp-zovldbkfz-oxyyfq-rpbo-qbpqfkd-367[foblp]\niqmbazulqp-dmnnuf-fqotzaxask-170[mnuiw]\nixccb-iorzhu-dftxlvlwlrq-439[katfr]\ngpsxdprixkt-uadltg-rdcipxcbtci-115[sxkct]\nnpmhcargjc-qaytclecp-fslr-pcqcypaf-990[soyhd]\nhqtyeqsjylu-uww-tufbeocudj-920[zlroy]\nclotzlnetgp-ojp-dezclrp-431[lpceo]\nwfummczcyx-wuhxs-lywycpcha-110[eatif]\njshzzpmplk-wshzapj-nyhzz-zavyhnl-643[zhpaj]\nhqtyeqsjylu-sqdto-seqjydw-bqrehqjeho-946[ltnyb]\neza-dpncpe-mfyyj-cplnbftdtetzy-717[oxwat]\nxmtjbzidx-xjgjmapg-ytz-mzvxlpdndodji-603[ksiqx]\nugdgjxmd-vqw-vwhsjlewfl-684[sxfvh]\nynssr-xzz-xgzbgxxkbgz-839[xzgbs]\ntagzsrsjvgmk-xdgowj-ljsafafy-918[agjsf]\nvrurcjah-pajmn-lqxlxujcn-uxprbcrlb-953[romck]\njshzzpmplk-qlssfilhu-bzly-alzapun-773[ojiwl]\npinovwgz-ytz-xjiovdihzio-655[yrfzp]\npualyuhapvuhs-yhiipa-thuhnltlua-903[hualp]\nhcd-gsqfsh-awzwhofm-ufors-dzoghwq-ufogg-fsgsofqv-870[yfizu]\nvrurcjah-pajmn-mhn-vjwjpnvnwc-563[rften]\nvkrhzxgbv-cxeeruxtg-ybgtgvbgz-215[lswez]\npkl-oaynap-lhwopey-cnwoo-hkceopeyo-316[opeya]\nbdavqofuxq-rxaiqd-ymzmsqyqzf-378[hguys]\nuqtqbizg-ozilm-ntwemz-wxmzibqwva-876[gzhyw]\njyddc-fyrrc-xvemrmrk-360[ulmzd]\njchipqat-rpcsn-rdpixcv-pcpanhxh-687[ltzwy]\ndfcxsqhwzs-xszzmpsob-hsqvbczcum-376[agmnj]\nvqr-ugetgv-gii-fgukip-856[giuve]\nxmtjbzidx-agjrzm-jkzmvodjin-811[wavdq]\nrmn-qcapcr-djmucp-sqcp-rcqrgle-756[sozba]\neadalsjq-yjsvw-tskcwl-suimakalagf-788[hmgzu]\ntinnm-qobrm-kcfygvcd-350[lzrje]\noxjmxdfkd-zelzlixqb-pqloxdb-965[xdlbo]\nhdgdovmt-bmvyz-ezggtwzvi-omvdidib-863[dvgim]\najyqqgdgcb-aylbw-amyrgle-cleglccpgle-522[ynhwt]\noazegyqd-sdmpq-ngzzk-fdmuzuzs-586[sygha]\nmyxcewob-qbkno-lexxi-oxqsxoobsxq-484[fmyeh]\npyknyegle-aylbw-amyrgle-mncpyrgmlq-470[dgahb]\nsehheiylu-hqrryj-huqsgkyiyjyed-972[apoin]\niutyaskx-mxgjk-hatte-iayzuskx-ykxboik-176[ctnms]\nuzfqdzmfuazmx-ngzzk-bgdotmeuzs-508[nslqc]\nnglmtuex-ktfitzbgz-wrx-kxvxbobgz-397[txgba]\ngbc-frperg-rtt-npdhvfvgvba-143[grvbf]\ntfejldvi-xiruv-wlqqp-avccpsvre-tfekrzedvek-815[cmtyq]\nchnylhuncihuf-wbiwifuny-lymyulwb-162[uyhil]\ndzczkrip-xiruv-gcrjkzt-xirjj-uvgrikdvek-113[hvwun]\nrgllk-ngzzk-emxqe-794[snuev]\nqvbmzvibqwvit-kivlg-zmkmqdqvo-876[ivunt]\ncqwdujys-fbqijys-whqii-ixyffydw-374[gcmut]\nsgmtkzoi-vrgyzoi-mxgyy-cuxqynuv-852[ygimo]\napuut-xcjxjgvoz-pnzm-oznodib-109[ozjnp]\nymszqfuo-gzefmnxq-ngzzk-fqotzaxask-326[zfqag]\nforwcoqhwjs-xszzmpsob-gsfjwqsg-610[rlhwt]\nvcibutulxiom-vohhs-xyjulngyhn-708[dypil]\nsgmtkzoi-inuiurgzk-jkbkruvsktz-124[qxmsb]\nluxciuwncpy-mwupyhayl-bohn-uhufsmcm-604[uotjd]\njyfvnlupj-kfl-bzly-alzapun-591[lafjn]\ndkqjcbctfqwu-hnqygt-ceswkukvkqp-622[skwtc]\nodiih-yujbcrl-pajbb-bcxajpn-771[otehb]\ndmbttjgjfe-gmpxfs-sftfbsdi-649[asqgv]\nvhglnfxk-zktwx-wrx-wxiehrfxgm-345[hipzg]\nncjzrpytn-ojp-xlcvpetyr-379[wuezq]\nykhknbqh-ywjzu-ykwpejc-opknwca-238[nxhwm]\nide-htrgti-gpqqxi-prfjxhxixdc-609[lhtnk]\ntinnm-qvcqczohs-hfowbwbu-272[xwhnz]\nkmjezxodgz-wvnfzo-hvivbzhzio-603[ftdkv]\nmolgbzqfib-mixpqfz-doxpp-ildfpqfzp-237[sodim]\ntmrszakd-okzrshb-fqzrr-kzanqzsnqx-287[zbmsl]\noxaflxzqfsb-mixpqfz-doxpp-abmilvjbkq-341[xbfpq]\nzuv-ykixkz-hatte-zxgototm-150[tzkox]\nytu-xjhwjy-kqtbjw-xmnuunsl-515[rbjpq]\noqnidbshkd-bzmcx-cdrhfm-183[dbchm]\nipvohghykvbz-ihzrla-zavyhnl-799[gdqfx]\npdjqhwlf-vfdyhqjhu-kxqw-uhdftxlvlwlrq-153[zqldc]\nkmjezxodgz-ytz-yzndbi-967[gierw]\ncvabijtm-rmttgjmiv-xczkpiaqvo-720[imtva]\nnglmtuex-ietlmbv-zktll-hixktmbhgl-215[nmwhy]\nvxupkizork-sorozgxe-mxgjk-lruckx-giwaoyozout-696[lkftj]\nmvhkvbdib-kgvnodx-bmvnn-xjiovdihzio-785[srjut]\neqnqthwn-rncuvke-itcuu-ewuvqogt-ugtxkeg-518[cfdqb]\nwfruflnsl-wfggny-htsyfnsrjsy-359[fsnvr]\niwcjapey-ywjzu-ykwpejc-nayaerejc-576[myaou]\nnsyjwsfyntsfq-kqtbjw-tujwfyntsx-593[swzqr]\nvhkkhlbox-ktwbhtvmbox-utldxm-mktbgbgz-501[yfqzw]\nqzoggwtwsr-rms-fsqswjwbu-324[grdjl]\ncybyjqho-whqtu-sqdto-seqjydw-ixyffydw-114[yqdwf]\nchnylhuncihuf-wfummczcyx-zfiqyl-guleyncha-136[jzbiq]\nzuv-ykixkz-jek-ykxboiky-904[mfadn]\nqjopwxha-sawlkjevaz-oywrajcan-dqjp-oanreyao-498[smtnr]\ndlhwvupglk-qlssfilhu-wbyjohzpun-695[lhups]\nudskkaxawv-usfvq-ugslafy-sfsdqkak-684[syldq]\ncybyjqho-whqtu-tou-huiuqhsx-582[dkbhi]\nbnqqnrhud-dff-kzanqzsnqx-833[dtzyw]\ntipfxvezt-upv-kvtyefcfxp-685[buszt]\napwmeclga-cee-qcptgacq-392[yszmf]\nzloolpfsb-pzxsbkdbo-erkq-pqloxdb-211[lykdq]\nlzfmdshb-tmrszakd-bzmcx-bnzshmf-qdrdzqbg-313[zbdms]\npbafhzre-tenqr-onfxrg-ratvarrevat-403[bktor]\npxtihgbsxw-vahvhetmx-mxvaghehzr-631[hxvae]\nvrurcjah-pajmn-ouxfna-jwjuhbrb-641[neckb]\npelbtravp-pubpbyngr-fnyrf-975[gndzm]\nvjpwncrl-mhn-jlzdrbrcrxw-485[zopte]\ndrxevkzt-sleep-uvgcfpdvek-945[bvnau]\nnzcczdtgp-mfyyj-dlwpd-613[yzbdk]\nyhwooebeaz-nwxxep-pnwejejc-238[ewjno]\nbuzahisl-msvdly-dvyrzovw-643[gbeat]\nqzlozfhmf-bzmcx-qdzbpthrhshnm-443[qosty]\nhvbizodx-zbb-adivixdib-343[nhyjs]\nfruurvlyh-lqwhuqdwlrqdo-gbh-vklsslqj-803[qpinz]\nkzgwomvqk-moo-twoqabqka-642[puwmb]\nibghopzs-foadouwbu-pogysh-hfowbwbu-480[rktvw]\nwsvsdkbi-qbkno-mkxni-nozkbdwoxd-588[wsytr]\nfkqbokxqflkxi-zxkav-abpfdk-263[kfxab]\nesyfwlau-jsttal-ogjckzgh-320[wufhe]\npxtihgbsxw-xzz-ehzblmbvl-319[nkcmq]\naflwjfslagfsd-bwddqtwsf-wfyafwwjafy-996[jkqhc]\nhafgnoyr-enoovg-phfgbzre-freivpr-429[xwuvb]\njlidywncfy-xsy-xyjulngyhn-916[zotqu]\ntfiifjzmv-gcrjkzt-xirjj-ivtvzmzex-971[cetnj]\nbnmrtldq-fqzcd-eknvdq-rsnqzfd-885[ektcl]\nluxciuwncpy-yaa-mniluay-266[auyci]\nhqfxxnknji-hmthtqfyj-wjhjnansl-801[zywic]\nvotubcmf-tdbwfohfs-ivou-efwfmpqnfou-129[foubm]\nthnulapj-jovjvshal-hjxbpzpapvu-253[ckgst]\nxlrypetn-mldvpe-lylwjdtd-457[lsmgz]\novbunmneqbhf-pnaql-svanapvat-351[alynm]\nrdchjbtg-vgpst-rpcsn-rdpixcv-detgpixdch-765[hptsq]\naczupnetwp-xtwtelcj-rclop-dnlgpyrpc-sfye-dstaatyr-899[onyrk]\nkrxqjijamxdb-kjbtnc-ldbcxvna-bnaerln-511[cyist]\noknkvcta-itcfg-tcddkv-fgukip-700[hycuv]\nkgjgrypw-epybc-zyqicr-mncpyrgmlq-288[ijbzo]\njyddc-hci-hizipstqirx-620[ervwu]\noknkvcta-itcfg-lgnnadgcp-ewuvqogt-ugtxkeg-544[mxano]\nvhglnfxk-zktwx-ktuubm-ftkdxmbgz-527[zfsoa]\nqcffcgwjs-rms-rsgwub-350[wstyq]\ntipfxvezt-treup-tfrkzex-uvgrikdvek-321[etkrv]\nlsyrkjkbnyec-lkcuod-nozkbdwoxd-874[kdobc]\nytu-xjhwjy-ojqqdgjfs-jslnsjjwnsl-437[nzycs]\nxjgjmapg-nxvqzibzm-cpio-yzkvmohzio-967[vasue]\nrkpqxyib-yxphbq-abpfdk-627[rvpcm]\nqyujihctyx-wuhxs-wiuncha-mylpcwym-604[ychuw]\nudglrdfwlyh-zhdsrqlchg-fdqgb-frqwdlqphqw-335[mtvzs]\nbnmrtldq-fqzcd-bgnbnkzsd-qdbdhuhmf-261[ywqhu]\nugfkmewj-yjsvw-tskcwl-dgyaklauk-996[kwagj]\niqmbazulqp-qss-pqbmdfyqzf-456[ztynb]\nawzwhofm-ufors-xszzmpsob-aofyshwbu-818[ycfar]\nwfintfhynaj-kqtbjw-qfgtwfytwd-411[ftwjn]\nnzydfxpc-rclop-dnlgpyrpc-sfye-opdtry-301[jwahc]\nyaxsnlcrun-snuuhknjw-bjunb-147[zsycg]\ncebwrpgvyr-qlr-fgbentr-923[xregt]\ntyepcyletzylw-mldvpe-opalcexpye-457[ebvtl]\npbeebfvir-onfxrg-phfgbzre-freivpr-299[refbp]\nvrurcjah-pajmn-npp-mnbrpw-953[hwayg]\nkzeed-wfggny-fhvznxnynts-775[bmnjw]\ntcorcikpi-ejqeqncvg-wugt-vguvkpi-336[cgive]\nmbiyqoxsm-mkxni-mykdsxq-crszzsxq-224[mgtde]\nbwx-amkzmb-kpwkwtibm-uizsmbqvo-616[zywgf]\nqfkkj-mldvpe-afcnsldtyr-925[dfkla]\nqzoggwtwsr-qobrm-qcbhowbasbh-974[vdxcz]\njshzzpmplk-yhiipa-bzly-alzapun-279[pzalh]\nzotts-vumeyn-mniluay-344[moyzn]\neza-dpncpe-nlyoj-nzletyr-dezclrp-249[rmlfn]\nrdadguja-ytaanqtpc-sthxvc-895[atcdg]\nbkzrrhehdc-rbzudmfdq-gtms-trdq-sdrshmf-729[vnaxm]\nwifilzof-willimcpy-vohhs-mniluay-864[rxqlk]\ndzczkrip-xiruv-zekvierkzferc-gcrjkzt-xirjj-uvmvcfgdvek-529[mautj]\nhafgnoyr-pelbtravp-onfxrg-erprvivat-741[xvymo]\nxmrrq-tskcwl-ksdwk-268[uzesm]\nhtsxzrjw-lwfij-kqtbjw-yjhmstqtld-801[jtwhl]\navw-zljyla-msvdly-yljlpcpun-435[cedbt]\nzovldbkfz-zxkav-zlxqfkd-xznrfpfqflk-185[fzklx]\ngvcskirmg-gerhc-wxsveki-308[gceik]\ngpsxdprixkt-snt-ldgzhwde-167[zbkqn]\ndkqjcbctfqwu-eqttqukxg-tcddkv-fgxgnqrogpv-466[eygsw]\nthnulapj-kfl-lunpullypun-643[zyucd]\nvjpwncrl-kjbtnc-mnenuxyvnwc-641[ncjvw]\nsgmtkzoi-atyzghrk-hgyqkz-xkykgxin-488[jyivp]\nzvyvgnel-tenqr-rtt-erprvivat-299[dvxye]\nvehmsegxmzi-gpewwmjmih-ikk-hizipstqirx-698[xtwpi]\nsno-rdbqds-lhkhszqx-fqzcd-bzmcx-bnzshmf-lzqjdshmf-287[twsqz]\njqwpihizlwca-zijjqb-lmdmtwxumvb-694[vhibn]\nfodvvlilhg-fkrfrodwh-wudlqlqj-595[ldfho]\nnuatmlmdpage-qss-efadmsq-248[kzgwp]\nsehheiylu-isqludwuh-xkdj-efuhqjyedi-894[ehudi]\nbpvctixr-hrpktcvtg-wjci-itrwcdadvn-843[gjtsq]\nsehheiylu-zubboruqd-tufbeocudj-556[ubedh]\npinovwgz-wvnfzo-gvwjmvojmt-291[spxor]\nvhkkhlbox-lvtoxgzxk-angm-kxlxtkva-163[kxlva]\nshmml-pubpbyngr-qrcyblzrag-273[xycpv]\nlahxpnwrl-mhn-anjlzdrbrcrxw-303[rlnah]\nvhglnfxk-zktwx-cxeeruxtg-wxlbzg-137[xhfpw]\nvagreangvbany-pnaql-svanapvat-845[anvgp]\nrzvkjiduzy-xviyt-xjvodib-gvwjmvojmt-655[ghens]\nygcrqpkbgf-ejqeqncvg-rwtejcukpi-388[xjiod]\nwlqqp-kfg-jvtivk-gcrjkzt-xirjj-tfekrzedvek-997[kjert]\nucynmlgxcb-djmucp-asqrmkcp-qcptgac-366[wqhry]\notzkxtgzoutgr-lruckx-ygrky-202[gtxfy]\nhoungfgxjuay-hgyqkz-ktmotkkxotm-748[kgoth]\nbnknqetk-bzmcx-kzanqzsnqx-989[nkqzb]\nvrurcjah-pajmn-mhn-lxwcjrwvnwc-251[jaxic]\nsbqiiyvyut-tou-efuhqjyedi-894[qksiu]\noaddaeuhq-bxmefuo-sdmee-efadmsq-716[inakb]\nvkrhzxgbv-wrx-phkdlahi-215[hkrvx]\nxcitgcpixdcpa-tvv-gtprfjxhxixdc-999[jemot]\nvehmsegxmzi-veffmx-wxsveki-594[bhgyq]\nlaffe-vrgyzoi-mxgyy-uvkxgzouty-124[ygfou]\nqzlozfhmf-dff-zbpthrhshnm-651[mkbun]\nxmrrq-wyy-dgyaklauk-138[yakrd]\ncvabijtm-kivlg-kwvbiqvumvb-980[vbikm]\nhmsdqmzshnmzk-azrjds-sdbgmnknfx-989[lvuhe]\nvdzonmhydc-dff-sqzhmhmf-625[enwxv]\npwcvonofrcig-xszzmpsob-gvwddwbu-740[hlvts]\nlnkfaypeha-oywrajcan-dqjp-ajcejaanejc-732[ajcen]\nugfkmewj-yjsvw-xdgowj-sfsdqkak-606[xnjmw]\nbqvvu-ywjzu-ykwpejc-opknwca-940[zywlu]\nvdzonmhydc-azrjds-zbpthrhshnm-131[dnjcy]\nvqr-ugetgv-fag-nqikuvkeu-544[sydvo]\nvjpwncrl-bljenwpna-qdwc-anbnjalq-693[najlw]\npbybeshy-fpniratre-uhag-ybtvfgvpf-481[msyze]\nyhwooebeaz-ynukcajey-xwogap-hkceopeyo-212[eoyac]\nyrwxefpi-hci-xiglrspskc-438[zytvr]\nujoon-tvv-hwxeexcv-427[ukymv]\nnsyjwsfyntsfq-wfggny-ijajqturjsy-957[pboys]\nzotts-vumeyn-lywycpcha-838[ujstb]\nupq-tfdsfu-dipdpmbuf-tijqqjoh-129[bluat]\noazegyqd-sdmpq-eomhqzsqd-tgzf-emxqe-170[yopas]\nktfitzbgz-vtgwr-vhtmbgz-kxtvjnblbmbhg-735[trlen]\nrdggdhxkt-uadltg-jhtg-ithixcv-401[yixqs]\nqfkkj-clmmte-opdtry-639[kmtcd]\nibghopzs-pibbm-rsdofhasbh-220[sutpe]\neqnqthwn-ecpfa-eqcvkpi-ocpcigogpv-596[qmfhp]\nhwdtljsnh-hfsid-htfynsl-zxjw-yjxynsl-931[nmojg]\nykjoqian-cnwza-xwogap-paydjkhkcu-472[akcjn]\nxlrypetn-nlyoj-nzletyr-opawzjxpye-197[fevmd]\nlzfmdshb-azrjds-kzanqzsnqx-755[zftaw]\napuut-xjgjmapg-xcjxjgvoz-mznzvmxc-577[gnzmx]\nhqcfqwydw-hqrryj-ijehqwu-608[qhwjr]\nlnkfaypeha-ejpanjwpekjwh-zua-pnwejejc-368[vwqni]\nbjfutsneji-jll-xmnuunsl-853[ozghw]\nmuqfedyput-ydjuhdqjyedqb-vbemuh-tulubefcudj-712[lqaik]\nwillimcpy-jlidywncfy-wuhxs-guhuaygyhn-214[itesx]\nrkpqxyib-zixppfcfba-ciltbo-rpbo-qbpqfkd-887[bpfiq]\neadalsjq-yjsvw-usfvq-ugslafy-ljsafafy-788[asfjl]\ngvaaz-kfmmzcfbo-qvsdibtjoh-103[ankyj]\nshmml-pnaql-pbngvat-phfgbzre-freivpr-403[mofch]\nshmml-cynfgvp-tenff-hfre-grfgvat-273[fgehm]\nibghopzs-tzcksf-difqvogwbu-870[bxgar]\nymszqfuo-rxaiqd-dqmocgueufuaz-196[xmwtu]\negdytrixat-uadltg-hidgpvt-115[mslhc]\nrkpqxyib-oxyyfq-abpfdk-445[qlrak]\nirdgrxzex-lejkrscv-irsszk-jkfirxv-191[izgye]\njsvagsulanw-hdsklau-yjskk-sfsdqkak-112[skadj]\nzgmfyxypbmsq-hcjjwzcyl-bctcjmnkclr-600[cjmyb]\njqwpihizlwca-ntwemz-uizsmbqvo-616[gijkn]\nguahyncw-wuhxs-wiuncha-nywbhifias-994[cipny]\nxgsvgmotm-kmm-ktmotkkxotm-436[ywzib]\nykhknbqh-ywjzu-zalwnpiajp-186[csbmn]\nudpsdjlqj-fkrfrodwh-zrunvkrs-283[rdfjk]\nyuxufmdk-sdmpq-eomhqzsqd-tgzf-mocgueufuaz-820[mskbl]\nsbqiiyvyut-isqludwuh-xkdj-qsgkyiyjyed-530[ndmuc]\nmbiyqoxsm-oqq-crszzsxq-952[gxqmn]\nrwcnawjcrxwju-lqxlxujcn-cnlqwxuxph-849[zqekt]\nkpvgtpcvkqpcn-fag-ugtxkegu-986[qpyuj]\ndfcxsqhwzs-qzoggwtwsr-qvcqczohs-fsoqeiwgwhwcb-714[lgtfc]\nojk-nzxmzo-xviyt-xjvodib-omvdidib-265[iodvx]\nwbhsfbohwcboz-qobrm-zcuwghwqg-298[bwhoc]\nshoewudys-tou-ixyffydw-478[uszty]" -> [w11]
    tunnel: [w10] -> w4 mode=indexing
    stop <- w9 stop-if-true
    n2 = Match Pattern(string=w11, regular expression="\n") -> (before substring=w10:string, after substring=w8:string)  [unwired: 1 in, 2 out]
    n3 = Equal?(x=w8, y="") -> (x = y?=w9:bool)
  }
  n4 = while {
    tunnel: w4 -> [w29] mode=indexing
    tunnel: [w15] -> w2 mode=indexing
    tunnel: [w12] -> w1
    i -> [w33]
    stop <- w32 stop-if-true
    n5 = Reverse String(1:w29) -> (0:w27:string)
    n6 = Match Pattern(string=w27, regular expression="-", offset (0)=10) -> (before substring=w24:string, after substring=w25:string)  [unwired: 2 out]
    n7 = Reverse String(1:w25) -> (0:w14:string)
    n8 = Reverse String(1:w24) -> (0:w21:string)
    n9 = Decimal String To Number(string=w21) -> (number=w13:i32)  [unwired: 2 in, 1 out]
    n10 = String Subset(string=w21, offset (0)=4, length (rest)=5 ("length (rest)")) -> (substring=w18:string)
    n11 = for {
      N: 26 -> [_]
      tunnel: w14 -> [w106]
      tunnel: [w77] -> w17
      i -> [w104]
      n12 = local read "CharPlusNombre"() -> (w103:i32[])
      n13 = local read "CharPlusLettre"() -> (w100:string[])
      n14 = Index Array(array=w103) -> (element #1=w92:i32, element #2=w91:i32, element #3=w90:i32, element #4=w89:i32, element #5=w88:i32)  [unwired: 5 in]
      n15 = Index Array(array=w100) -> (element #1=w87:string, element #2=w86:string, element #3=w85:string, element #4=w84:string, element #5=w83:string)  [unwired: 5 in]
      n16 = Index Array(array=string[] ["a", "b", "c", "d", "e", "f", "g", "h", "i", "j", "k", "l", "m", "n", "o", "p", "q", "r", "s", "t", "u", "v", "w", "x", "y", "z"], index=w104) -> (element=w101:string)
      n17 = Search and Replace String(replace all?=TRUE ("replace all? (F)"), input string=w106, search string=w101) -> (number of replacements=w102:i32)  [unwired: 5 in, 3 out]
      n18 = while {
        tunnel: w102 -> [w112]
        tunnel: w101 -> [w132]
        shift-right: [w131] -> w82
        shift-left: w87 -> [w129]
        shift-right: [w133] -> w97
        shift-left: w92 -> [w130]
        shift-right: [w125] -> w78
        shift-left: w83 -> [w128]
        shift-right: [w123] -> w79
        shift-left: w84 -> [w124]
        shift-right: [w126] -> w80
        shift-left: w85 -> [w127]
        shift-right: [w121] -> w81
        shift-left: w86 -> [w122]
        shift-right: [w115] -> w96
        shift-left: w91 -> [w116]
        shift-right: [w113] -> w95
        shift-left: w90 -> [w114]
        shift-right: [w119] -> w94
        shift-left: w89 -> [w120]
        shift-right: [w117] -> w93
        shift-left: w88 -> [w118]
        i -> [w107]
        stop <- w110 stop-if-true
        n19 = case shown="0, Default" w107 {
          tunnel: [w157 w203 w249 w295 w341] -> w133
          tunnel: w132 -> [w156 w202 w248 w294 w340]
          tunnel: [w155 w201 w247 w293 w339] -> w131
          tunnel: w130 -> [w134 w181 w228 w274 w320]
          tunnel: w129 -> [w154 w200 w246 w292 w338]
          tunnel: [w153 w199 w245 w291 w337] -> w108
          tunnel: w128 -> [w152 w198 w244 w290 w336]
          tunnel: w127 -> [w151 w197 w243 w289 w335]
          tunnel: [w150 w196 w242 w288 w334] -> w126
          tunnel: [w149 w195 w241 w287 w333] -> w125
          tunnel: w124 -> [w148 w194 w240 w286 w332]
          tunnel: [w147 w193 w239 w285 w331] -> w123
          tunnel: w122 -> [w146 w192 w238 w284 w330]
          tunnel: [w145 w191 w237 w283 w329] -> w121
          tunnel: w120 -> [w144 w190 w236 w272 w328]
          tunnel: [w143 w189 w235 w282 w327] -> w119
          tunnel: w118 -> [w142 w188 w234 w281 w318]
          tunnel: [w141 w187 w233 w280 w326] -> w117
          tunnel: w116 -> [w140 w180 w227 w273 w319]
          tunnel: [w139 w186 w232 w279 w325] -> w115
          tunnel: w114 -> [w138 w185 w226 w278 w324]
          tunnel: [w137 w184 w231 w277 w323] -> w113
          tunnel: w112 -> [w135 w182 w229 w275 w321]
          frame 0, Default {
            n20 = Greater?(x=w135, y=w134) -> (0:w136:bool)
            n21 = case shown="True" w136 {
              tunnel: [w167 w174] -> w157
              tunnel: w156 -> [_ w169]
              tunnel: w154 -> [w158 w179]
              tunnel: [w158 w169] -> w155
              tunnel: [FALSE TRUE] -> w153
              tunnel: w152 -> [w162 _]
              tunnel: w134 -> [w167 w175]
              tunnel: w151 -> [w160 w177]
              tunnel: [w160 w176] -> w150
              tunnel: [w162 w178] -> w149
              tunnel: w148 -> [w161 w178]
              tunnel: [w161 w177] -> w147
              tunnel: w146 -> [w159 w176]
              tunnel: [w159 w179] -> w145
              tunnel: w144 -> [w164 w171]
              tunnel: [w164 w172] -> w143
              tunnel: w142 -> [w163 _]
              tunnel: [w163 w171] -> w141
              tunnel: w140 -> [w166 w173]
              tunnel: [w166 w175] -> w139
              tunnel: w138 -> [w165 w172]
              tunnel: [w165 w173] -> w137
              tunnel: w135 -> [_ w174]
              frame False {
              }
              frame True {
              }
            }
          }
          frame 1 {
            n22 = Greater?(x=w182, y=w180) -> (0:w183:bool)
            n23 = case shown="True" w183 {
              tunnel: [w213 w217] -> w203
              tunnel: w202 -> [_ w218]
              tunnel: w200 -> [w204 w219]
              tunnel: [w204 w219] -> w201
              tunnel: [FALSE TRUE] -> w199
              tunnel: w198 -> [w208 _]
              tunnel: w181 -> [w213 w217]
              tunnel: w197 -> [w206 w224]
              tunnel: [w206 w223] -> w196
              tunnel: [w208 w225] -> w195
              tunnel: w194 -> [w207 w225]
              tunnel: [w207 w224] -> w193
              tunnel: w192 -> [w205 w223]
              tunnel: [w205 w218] -> w191
              tunnel: w190 -> [w210 w215]
              tunnel: [w210 w221] -> w189
              tunnel: w188 -> [w209 _]
              tunnel: [w209 w215] -> w187
              tunnel: w180 -> [w212 w222]
              tunnel: [w212 w216] -> w186
              tunnel: w185 -> [w211 w221]
              tunnel: [w211 w222] -> w184
              tunnel: w182 -> [_ w216]
              frame False {
              }
              frame True {
              }
            }
          }
          frame 2 {
            n24 = Greater?(x=w229, y=w226) -> (0:w230:bool)
            n25 = case shown="True" w230 {
              tunnel: [w259 w266] -> w249
              tunnel: w248 -> [_ w264]
              tunnel: w246 -> [w250 w267]
              tunnel: [w250 w267] -> w247
              tunnel: [FALSE TRUE] -> w245
              tunnel: w244 -> [w254 _]
              tunnel: w228 -> [w259 w266]
              tunnel: w243 -> [w252 w270]
              tunnel: [w252 w264] -> w242
              tunnel: [w254 w271] -> w241
              tunnel: w240 -> [w253 w271]
              tunnel: [w253 w270] -> w239
              tunnel: w238 -> [w251 w263]
              tunnel: [w251 w263] -> w237
              tunnel: w236 -> [w256 w265]
              tunnel: [w256 w269] -> w235
              tunnel: w234 -> [w255 _]
              tunnel: [w255 w265] -> w233
              tunnel: w227 -> [w258 w261]
              tunnel: [w258 w261] -> w232
              tunnel: w226 -> [w257 w269]
              tunnel: [w257 w262] -> w231
              tunnel: w229 -> [_ w262]
              frame False {
              }
              frame True {
              }
            }
          }
          frame 3 {
            n26 = Greater?(x=w275, y=w272) -> (0:w276:bool)
            n27 = case shown="True" w276 {
              tunnel: [w305 w314] -> w295
              tunnel: w294 -> [_ w308]
              tunnel: w292 -> [w296 w315]
              tunnel: [w296 w315] -> w293
              tunnel: [FALSE TRUE] -> w291
              tunnel: w290 -> [w300 _]
              tunnel: w274 -> [w305 w314]
              tunnel: w289 -> [w298 w307]
              tunnel: [w298 w307] -> w288
              tunnel: [w300 w317] -> w287
              tunnel: w286 -> [w299 w317]
              tunnel: [w299 w308] -> w285
              tunnel: w284 -> [w297 w312]
              tunnel: [w297 w312] -> w283
              tunnel: w272 -> [w302 w313]
              tunnel: [w302 w310] -> w282
              tunnel: w281 -> [w301 _]
              tunnel: [w301 w313] -> w280
              tunnel: w273 -> [w304 w311]
              tunnel: [w304 w311] -> w279
              tunnel: w278 -> [w303 w309]
              tunnel: [w303 w309] -> w277
              tunnel: w275 -> [_ w310]
              frame False {
              }
              frame True {
              }
            }
          }
          frame 4 {
            n28 = Greater?(x=w321, y=w318) -> (0:w322:bool)
            n29 = case shown="True" w322 {
              tunnel: [w351 w361] -> w341
              tunnel: w340 -> [_ w354]
              tunnel: w338 -> [w342 w362]
              tunnel: [w342 w362] -> w339
              tunnel: [FALSE TRUE] -> w337
              tunnel: w336 -> [w346 _]
              tunnel: w320 -> [w351 w361]
              tunnel: w335 -> [w344 w357]
              tunnel: [w344 w357] -> w334
              tunnel: [w346 w354] -> w333
              tunnel: w332 -> [w345 w353]
              tunnel: [w345 w353] -> w331
              tunnel: w330 -> [w343 w360]
              tunnel: [w343 w360] -> w329
              tunnel: w328 -> [w348 w355]
              tunnel: [w348 w355] -> w327
              tunnel: w318 -> [w347 _]
              tunnel: [w347 w356] -> w326
              tunnel: w319 -> [w350 w359]
              tunnel: [w350 w359] -> w325
              tunnel: w324 -> [w349 w358]
              tunnel: [w349 w358] -> w323
              tunnel: w321 -> [_ w356]
              frame False {
              }
              frame True {
              }
            }
          }
        }
        n30 = Equal?(x=w107, y=4) -> (x = y?=w109:bool)
        n31 = Or(x=w108, y=w109) -> (x .or. y?=w110:bool)
      }
      n32 = Build Array(w97, w96, w95, w94, w93) -> (w98:i32[])
      n33 = Build Array(w82, w81, w80, w79, w78) -> (w99:string[])
      n34 = Concatenate Strings(w82, w81, w80, w79, w78) -> (w77:string)
      n35 = local write "CharPlusNombre"(w98) -> ()
      n36 = local write "CharPlusLettre"(w99) -> ()
    }
    n37 = Equal?(x=w18, y=w17) -> (x = y?=w16:bool)
    n38 = case shown="True" w16 {
      tunnel: ["" w41] -> w15
      tunnel: w14 -> [_ w42]
      tunnel: w13 -> [_ w36]
      tunnel: [w34 w40] -> w12
      frame False {
        n39 = local read "Partie 2 ID"() -> (w34:i32)
      }
      frame True {
        w38 = "northpole" ("regular expression")
        n40 = Quotient & Remainder(x=w36, y=26) -> (x-y*floor(x/y)=w44:i32)  [unwired: 1 out]
        n41 = while {
          shift-right: [w64] -> _
          shift-left: w42 -> [w65]
          tunnel: w44 -> [w60]
          shift-right: [w58] -> w41
          shift-left: "" -> [w57]
          stop <- w63 stop-if-true
          w49 = 27 ("y")
          n42 = String Subset(string=w65, length (rest)=1 ("length (rest)")) -> (substring=w61:string)  [unwired: 1 in]
          n43 = while {
            tunnel: string[] ["a", "b", "c", "d", "e", "f", "g", "h", "i", "j", "k", "l", "m", "n", "o", "p", "q", "r", "s", "t", "u", "v", "w", "x", "y", "z", "", "-"] -> [w71] mode=indexing
            tunnel: w61 -> [w72]
            tunnel: [w69] -> w52
            i -> [w69]
            stop <- w70 stop-if-true
            n44 = Equal?(x=w72, y=w71) -> (x = y?=w70:bool)
          }
          n45 = Add(x=w60, y=w52) -> (x+y=w55:i32)
          n46 = Equal?(x=w52, y=w49) -> (x = y?=w53:bool)
          n47 = Quotient & Remainder(x=w55, y=26) -> (x-y*floor(x/y)=w51:i32)  [unwired: 1 out]
          n48 = case shown="True" w53 {
            tunnel: w51 -> [w67 _]
            tunnel: [w67 w68] -> w50
            tunnel: w49 -> [_ w68]
            frame False {
            }
            frame True {
            }
          }
          n49 = Index Array(array=string[] ["a", "b", "c", "d", "e", "f", "g", "h", "i", "j", "k", "l", "m", "n", "o", "p", "q", "r", "s", "t", "u", "v", "w", "x", "y", "z", "", "  "], index=w50) -> (element=w59:string)
          n50 = Match Pattern(string=w65, regular expression=w61) -> (after substring=w64:string)  [unwired: 1 in, 3 out]
          n51 = Equal?(x=w61, y="") -> (x = y?=w63:bool)
          n52 = Concatenate Strings(w57, w59) -> (w58:string)
        }
        n53 = Match Pattern(string=w41, regular expression=w38) -> (match substring=w37:string)  [unwired: 1 in, 3 out]
        n54 = Equal?(x=w38, y=w37) -> (x = y?=w39:bool)
        n55 = case shown="True" w39 {
          tunnel: w36 -> [_ w47]
          tunnel: [w46 w47] -> w40
          frame False {
            n56 = local read "Partie 2 ID"() -> (w46:i32)
          }
          frame True {
          }
        }
      }
    }
    n57 = case shown="True" w16 {
      tunnel: w13 -> [_ w75]
      frame False {
      }
      frame True {
        n58 = local read "Partie 1"() -> (w74:i32)
        n59 = Add(x=w75, y=w74) -> (x+y=w73:i32)
        n60 = local write "Partie 1"(w73) -> ()
      }
    }
    n61 = Equal?(x=w33, y=936) -> (x = y?=w32:bool)
    "CharPlusNombre" <- i32[] [-1, -1, -1, -1, -1] ("CharPlus")
    "CharPlusLettre" <- string[] [" ", " ", "", " ", " "] ("CharPlusLettre")
  }
  "Partie 2" <- w2
  "Partie 2 ID" <- w1
  "Partie 1" <- 0 ("number")
